vi "Copy State Data.vi"(8 "error in (no error)":errorcluster, 11 "State Machine in":refnum<class "State Machine.lvclass">) -> (0 "error out":errorcluster, 3 "State Machine out":refnum<class "State Machine.lvclass">)   [LabVIEW 2024]
uses:
  State Machine.lvclass
  State Machine.lvclass/State Machine.ctl
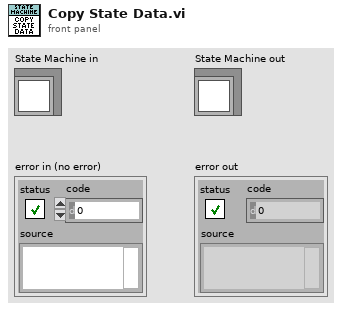
[diagram p1: front panel]
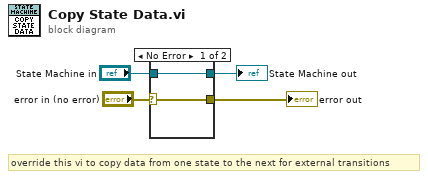
[diagram p0: block diagram]
diagram:
  # "override this vi to copy data from one state to the next for external transitions"
  n1 = case shown="No Error" "error in (no error)" {
    selector: "error in (no error)" -> [w5 w8]
    tunnel: [w5 w8] -> w3
    tunnel: [w6 w7] -> w1
    tunnel: "State Machine in" -> [w6 w7]
    frame No Error {
    }
    frame Error {
    }
  }
  "error out" <- w3
  "State Machine out" <- w1
